vi "final.vi"() -> ()   [LabVIEW 2024]
panel:
  out "2D Picture 2":picture
  in  "L 2":dbl(slide)=80.0 scale=0.0..200.0
  in  "L 1":dbl(slide)=80.0 scale=0.0..200.0
  in  "file (use dialog)":path
  in  "Timeout (ms)":u32=1000
  in  "VISA Refnum in":refnum<visa-resource-name>
  out "end effector":cluster{dbl, dbl}={159.01647214211073, 1.9100783062530127} {"?" format="%.1f"; "?" format="%#.1f"}
  out "2D Picture":picture
  in  "2D Pict origin":cluster{"x":dbl, "y":dbl}={"x"=200.0, "y"=200.0}
  # "mm"
  # "mm"
  # "mm"
  # "mm"
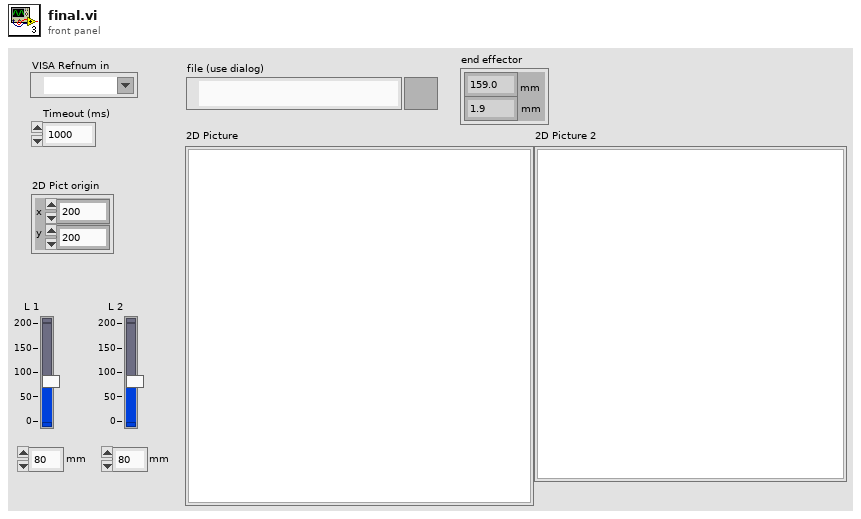
[diagram p1: front panel]
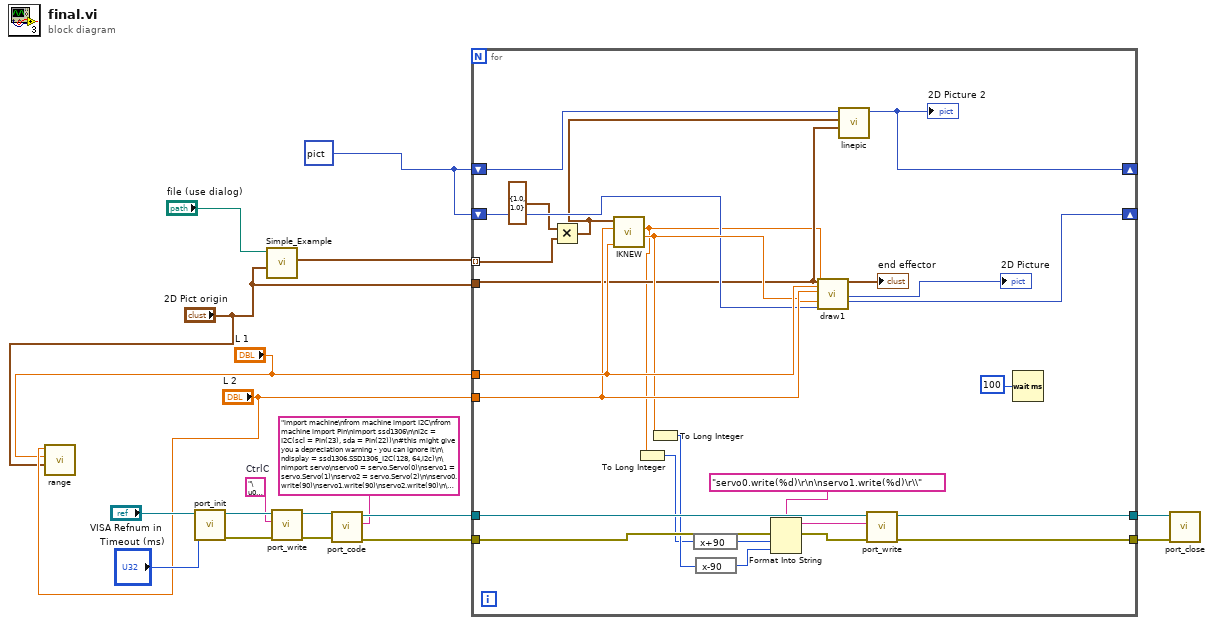
[diagram p0: block diagram]
diagram:
  w1 = picture data[5B] ("new picture")
  w11 = "\u0003"  # CtrlC
  n1 = call "range.vi"("2D Pict origin"="2D Pict origin", "L 1"="L 1", "L 2"="L 2") -> ()  [unwired: 8 in, 1 out]
  n2 = call <userlib>:"port_init.vi"("Timeout (ms)"="Timeout (ms)", "VISA Refnum in"="VISA Refnum in") -> ("error out"=w14:errorcluster, "VISA Refnum out"=w15:refnum<visa-resource-name>)  [unwired: 8 in]
  n3 = call <userlib>:"Simple_Example.vi"("2D Pict origin"="2D Pict origin", "file (use dialog)"="file (use dialog)") -> ("xy coord"=w18:cluster{"x":dbl, "y":dbl}[])  [unwired: 8 in, 1 out]
  n4 = call <userlib>:"port_write.vi"("error in (no error)"=w14, "write buffer"=w11, "VISA Refnum in"=w15) -> ("error out"=w12:errorcluster, "VISA Refnum out"=w13:refnum<visa-resource-name>)  [unwired: 7 in]
  n5 = call <userlib>:"port_code.vi"("error in (no error)"=w12, "Code to run"="import machine\nfrom machine import I2C\nfrom machine import Pin\nimport ssd1306\n\ni2c = I2C(scl = Pin(23), sda = Pin(22))\n#this might give you a depreciation warning - you can ignore it\n\ndisplay = ssd1306.SSD1306_I2C(128, 64,i2c)\n\nimport servo\nservo0 = servo.Servo(0)\nservo1 = servo.Servo(1)\nservo2 = servo.Servo(2)\n\nservo0.write(90)\nservo1.write(90)\nservo2.write(90)\n\ndisplay.rect(10,10,60,50,1)\ndisplay.text('Good Morning', 0, 0, 1)\ndisplay.show()\n    ", "VISA Refnum in"=w13) -> ("error out"=w9:errorcluster, "VISA Refnum out"=w10:refnum<visa-resource-name>)  [unwired: 7 in]
  n6 = for {
    tunnel: w18 -> [w28] mode=indexing
    tunnel: w10 -> [w41]
    tunnel: w9 -> [w43]
    tunnel: [w39] -> w7
    tunnel: [w38] -> w6
    tunnel: "2D Pict origin" -> [w26]
    shift-right: [w30] -> _
    shift-left: w1 -> [w32]
    shift-right: [w19] -> _
    shift-left: w1 -> [w37]
    tunnel: "L 1" -> [w35]
    tunnel: "L 2" -> [w34]
    n7 = Multiply(x=cluster{dbl, dbl} {1.0, 1.0}, y=w28) -> (x*y=w27:cluster{dbl, dbl})
    n8 = call "IKNEW.vi"("L1"=w35, "L2"=w34, "coordinates"=w27) -> ("theta21"=w33:dbl, "theta11"=w25:dbl)  [unwired: 7 in]
    n9 = To Long Integer(number=w25) -> (32bit integer=w22:i32)
    n10 = To Long Integer(number=w33) -> (32bit integer=w23:i32)
    n11 = expression code="x+90"(w22) -> (w21:i32)
    n12 = expression code="x-90"(w23) -> (w20:i32)
    n13 = Format Into String(format string="servo0.write(%d)\r\n\nservo1.write(%d)\r\\", error in=w43, w21, w20) -> (resulting string=w24:string, error out=w42:errorcluster)  [unwired: 1 in]
    n14 = call "draw1.vi"("new position"=w26, "L 1"=w35, "L 2"=w34, "Angle1"=w25, "Angle 2"=w33, "input pic in loop"=w32) -> ("end effector"=→"end effector":cluster{dbl, dbl}, "2D Picture"=→"2D Picture":picture, "shift pic"=w30:picture)  [unwired: 9 in, 2 out]
    n15 = call "linepic.vi"("origin"=w26, "Cluster"=w27, "shift pic"=w37) -> ("2D Picture 2"=w19:picture)  [unwired: 8 in]
    "2D Picture 2" <- w19
    n16 = call <userlib>:"port_write.vi"("error in (no error)"=w42, "write buffer"=w24, "VISA Refnum in"=w41) -> ("error out"=w38:errorcluster, "VISA Refnum out"=w39:refnum<visa-resource-name>)  [unwired: 7 in]
    n17 = Wait (ms)(milliseconds to wait=u32 100) -> ()  [unwired: 1 out]
  }
  n18 = call <userlib>:"port_close.vi"("error in (no error)"=w6, "VISA Refnum in"=w7) -> ()  [unwired: 10 in]
